vi "Get Name.vi"(11 "CD Template":refnum<class "NIVS_PPLCD Template.lvclass">) -> (2 "String":string)   [LabVIEW 2020, in "NIVS_PPLCD Template.lvclass"]
uses:
  NIVS_PPLCD Template.lvclass
  NIVS_CD Template/NIVS_CD Template.lvclass
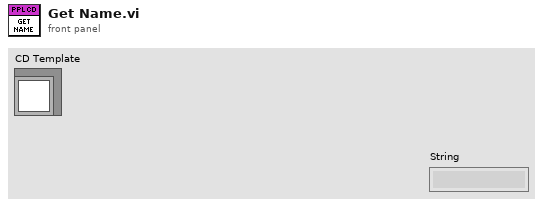
[diagram p1: front panel]
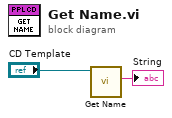
[diagram p0: block diagram]
diagram:
  n1 = call-parent "Get Name.vi"("CD Template"="CD Template") -> ("String"=→"String":string)  [unwired: 10 in]
